vi "Flatten.vi"(8 "error in (no error)":errorcluster, 10 "Pretty Print?":bool, 11 "JSON Object in":refnum<class "JSON Object.lvclass">) -> (0 "error out":errorcluster, 2 "String":string)   [LabVIEW 2011, in "JSON Object.lvclass"]
doc: "Converts an <b>JSON Object</b> into <b>String</b>. Use <b>Pretty Print?</b> to auto-indent and distribute the string over different lines.\n\nCopyright 2012 James David Powell, Shaun Rumbell and Ton Plomp\nMore information on http://lavag.org/topic/16217-cr-json-labview"
uses:
  JSON Object.lvclass
  JSON Object.lvclass/JSON Object.ctl
  JSON Value/JSON Value.lvclass
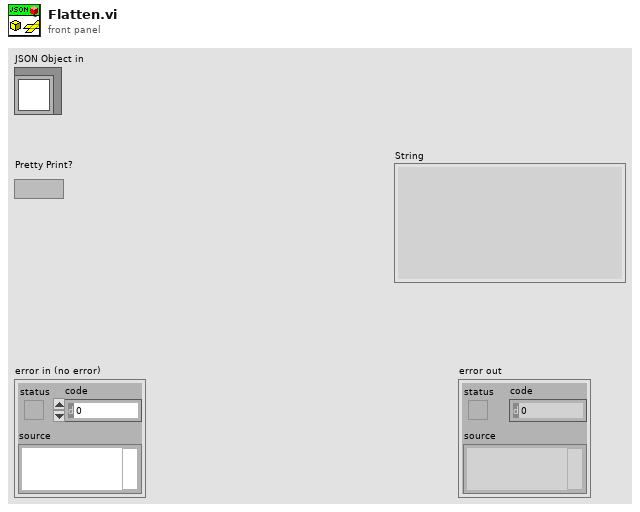
[diagram p1: front panel]
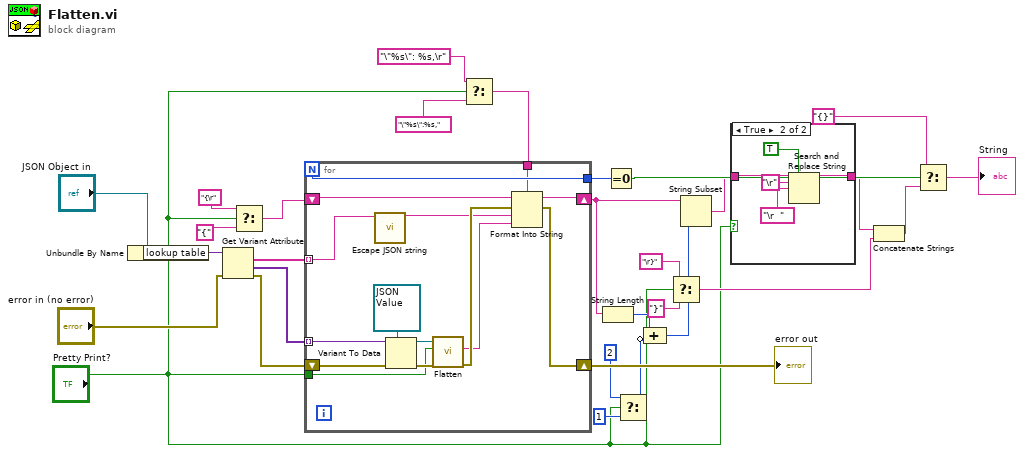
[diagram p0: block diagram]
diagram:
  n1 = Unbundle By Name("JSON Object in") -> ("lookup table"=w29:variant)
  n2 = Get Variant Attribute(Variant=w29, error in="error in (no error)") -> (names=w28:string[], values=w27:variant[], error out=w25:errorcluster)  [unwired: 2 in, 1 out]
  n3 = Select(t="{\r", s="Pretty Print?", f="{") -> (s? t:f=w16:string)
  n4 = Select(t="\"%s\": %s,\r" ("format string"), s="Pretty Print?", f="\"%s\":%s," ("format string")) -> (s? t:f=w5:string)
  n5 = for {
    N -> [w36]
    tunnel: w28 -> [w32] mode=indexing
    tunnel: w27 -> [w45] mode=indexing
    shift-right: [w37] -> w18
    shift-left: w16 -> [w42]
    shift-right: [w38] -> w24
    shift-left: w25 -> [w41]
    tunnel: [w36] -> w23
    tunnel: "Pretty Print?" -> [w35]
    tunnel: w5 -> [w33]
    n6 = call "Escape JSON string.vi"("Text (unscaped)"=w32) -> ("Text (escaped)"=w31:string)  [unwired: 9 in, 1 out]
    n7 = Variant To Data(error in=w41, type=refnum<class "JSON Value.lvclass"> refnum ("JSON Value.lvclass"), Variant=w45) -> (data=w43:refnum<class "JSON Value.lvclass">, error out=w40:errorcluster)
    n8 = call-dynamic "Flatten.vi"("error in (no error)"=w40, "Pretty Print?"=w35, "JSON Value in"=w43) -> ("error out"=w39:errorcluster, "String"=w34:string)  [unwired: 7 in]
    n9 = Format Into String(format string=w33, initial string=w42, error in=w39, w31, w34) -> (resulting string=w37:string, error out=w38:errorcluster)
  }
  "error out" <- w24
  n10 = String Length(string=w18) -> (length=w19:i32)
  n11 = Equal To 0?(x=w23) -> (x = 0?=w22:bool)
  n12 = Select(t=2, s="Pretty Print?", f=1) -> (s? t:f=w1:i32)
  n13 = Compound Arithmetic op=ADD(w19, invert w1) -> (w17:i32)
  n14 = Select(t="\r}" ("substring (\"\")"), s="Pretty Print?", f="}" ("substring (\"\")")) -> (s? t:f=w13:string)
  n15 = String Subset(string=w18, length (rest)=w17) -> (substring=w11:string)  [unwired: 1 in]
  n16 = case shown="True" "Pretty Print?" {
    tunnel: w11 -> [w46 w51]
    tunnel: [w46 w50] -> w10
    frame False {
    }
    frame True {
      n17 = Search and Replace String(replace all?=TRUE ("replace all? (F)"), input string=w51, search string="\r", replace string="\r  " ("search string")) -> (result string=w50:string)  [unwired: 4 in, 3 out]
    }
  }
  n18 = Concatenate Strings(w10, w13) -> (w9:string)
  n19 = Select(t="{}", s=w22, f=w9) -> (s? t:f=→"String":string)
